vi "Periodic Tasks.vi"(8 "error in (no error)":errorcluster) -> ()   [LabVIEW 2016]
doc: "This VI runs in parallel to other tasks. It can contain as many user-defined periodic loops as you need. These can carry out PID or other sorts of timed response."
uses:
  Extra/Global_Var-RefNum/Global_Var_Other.vi
  Extra/General/ArbitorSpecializations/Arbitor_Int.vi
  Extra/General/ArbitorSpecializations/Arbitor_Float.vi
  Extra/General/ArbitorSpecializations/Arbitor_Bool.vi
  Extra/Sensors/ADI MXP IMU/ADIS16448_IMU.lvlib
  Extra/Sensors/PixyCam/PixyCam_LabVIEW.lvlib
panel:
  in  "Manual_Gate_Control":enum16{"Stop", "Catch", "Clamp", "Open"}(ring)
  in  "Gear_Beam_Break_Sensor_Triggered":bool
  in  "RailOffset":dbl=5.0 format="%#_13g"
  in  "UltrasonicPercent":dbl=0.2
  in  "MaxRange":dbl=27.0
  out "Distance":dbl=15.697590634880541
  in  "GearRailWantedPosition":dbl(slide)=5.0 scale=5.0..25.0
  in  "GearRailPID":T1={"proportional gain (Kc)"=0.2, "integral time (Ti, min)"=0.0, "derivative time (Td, min)"=0.0001} {"derivative time (Td, min)" format="%.3g"; "integral time (Ti, min)" format="%.3g"; "proportional gain (Kc)" format="%.3g"}
  in  "ResetGearCollect":bool
  in  "ResetGearPlacer":bool
  in  "StartGearPlace":bool
  in  "Place":bool
  in  "Collect":bool
  in  "Manual":bool=TRUE
  in  "StartGearCollect":bool
  out "GateReached":bool
  in  "Drive PID Gains":T1={"proportional gain (Kc)"=0.04, "integral time (Ti, min)"=0.025, "derivative time (Td, min)"=1e-05}
  out "IMU Angles Out":T2={"X Angle"=24.903333526419914, "Y Angle"=134.91891868799198, "Z Angle"=-74.78372775360221}
  # "1/24/17 (2014 Chassis)\nKc=0.015\nTi=5\nTd=0.0005\nTurns slowly, but well"
  # "2014 Chassis\nKc=0.09\nTi=0.9\nTd=0.001\nNot good for turning"
  # "2/12/17 (2017 Chassis)\nKc= 0.04\nTi=.025\nTd=1E-5\ndrives straight"
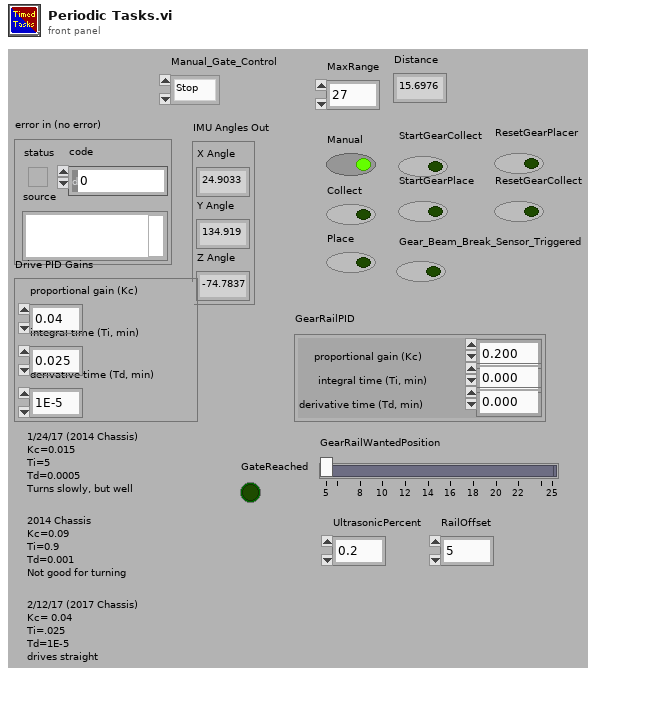
[diagram p1: front panel]
types:
  T1 = cluster{"proportional gain (Kc)":dbl, "integral time (Ti, min)":dbl, "derivative time (Td, min)":dbl}
  T2 = cluster{"X Angle":dbl, "Y Angle":dbl, "Z Angle":dbl}
  T3 = typedef "WPI_RobotDriveDevRef.ctl" = cluster{"DevStatus":errorcluster, "Motors[]":T4[], "Square Inputs":bool, "Max Output":dbl}
  T4 = typedef "WPI_MotorControlDeviceRef.ctl" = cluster{"DeviceStatus":errorcluster, "Type":T5, "PWM":cluster{"PWM Channel":T6, "DeadBand":T7}, "CAN":cluster{"Device Number":u8, "SetOutput VI Ref":variant, "GetOutput VI Ref":variant, "Enable VI Ref":variant, "Disable VI Ref":variant, "Data":variant}, "Invert":bool}
  T5 = typedef "WPI_MotorControlType.ctl" = enum16{"PWM", "CAN"}
  T6 = typedef "FPGA_DIOPWMChannel.ctl" = enum8{"PWM 0", "PWM 1", "PWM 2", "PWM 3", "PWM 4", "PWM 5", "PWM 6", "PWM 7", "PWM 8", "PWM 9", "PWM MXP 0", "PWM MXP 1", "PWM MXP 2", "PWM MXP 3", "PWM MXP 4", "PWM MXP 5", "PWM MXP 6", "PWM MXP 7", "PWM MXP 8", "PWM MXP 9", "Invalid"}
  T7 = typedef "WPI_PWMDeadband.ctl" = cluster{"Name":string, "maxPositivePwm":i32, "minPositivePwm":i32, "centerPwm":i32, "maxNegativePwm":i32, "minNegativePwm":i32, "angularRange":u16}
  T8 = typedef "PixyCam_LabVIEW.lvlib/PixyCam_DevRef.ctl" = cluster{"PixyCamDevRef_SPI":T9, "Communication Mode":T12, "Error":errorcluster}
  T9 = typedef "PixyCam_LabVIEW.lvlib/PixyCam_SPI_DevRef.ctl" = cluster{"SPIDevRef":T10, "Output Queue":refnum<queue>}
  T10 = typedef "WPI_SPIDevRef.ctl" = cluster{"DevStatus":errorcluster, "Handle":i32, "SPI Bus":T11}
  T11 = typedef "spi_bus.ctl" = enum16{"SPI On-Board, CS0", "SPI On-Board, CS1", "SPI On-Board, CS2", "SPI On-Board, CS3", "SPI MXP", "Invalid"}
  T12 = typedef "PixyCam_LabVIEW.lvlib/PixyCam_CommMode.ctl" = enum16{"SPI", "I2C", "UART", "Analog", "Digital"}
  T13 = typedef "ADIS16448_IMU.lvlib/ADI_IMU_ADIS16448_InterruptDevRef.ctl" = cluster{"ADI IMU DevRef":T14, "InterruptRef":T15}
  T14 = typedef "ADIS16448_IMU.lvlib/ADI_IMU_ADIS16448_IMUDevRef.ctl" = cluster{"DevStatus":errorcluster, "Handle":i32, "SPI Bus":T11, "Device Found":bool, "Device Ready":bool, "Yaw Axis":enum16{"X", "Y", "Z"}, "AHRS Algorithm":enum16{"Complementary", "Madgwick"}, "Serial":u16, "Lot ID 2":u16, "Lot ID 1":u16, "Product ID":u16}
  T15 = typedef "WPI_InterruptRef.ctl" = cluster{"DevStatus":errorcluster, "InterruptIndex":T16}
  T16 = typedef "FPGA_InterruptIndex.ctl" = enum8{"0", "1", "2", "3", "4", "5", "6", "7", "Invalid"}
  T17 = typedef "WPI_AnalogChannelDevRef.ctl" = cluster{"DevStatus":errorcluster, "Analog Channel":T18}
  T18 = typedef "FPGA_AIChannel.ctl" = enum8{"AI 0", "AI 1", "AI 2", "AI 3", "AI MXP 0", "AI MXP 1", "AI MXP 2", "AI MXP 3", "Invalid"}
  T19 = typedef "WPI_SonarMB1010DigitalDeviceRef.ctl" = cluster{"CounterDevRef":T20, "Scaling factor (s/in)":dbl}
  T20 = typedef "WPI_CounterDevRef.ctl" = cluster{"DevStatus":errorcluster, "CntIndex":T21}
  T21 = typedef "FPGA_CounterCtrSystemIndex.ctl" = enum8{"Ctr 0", "Ctr 1", "Ctr 2", "Ctr 3", "Ctr 4", "Ctr 5", "Ctr 6", "Ctr 7", "Invalid"}
  T22 = typedef "WPI_EncoderDevRef.ctl" = cluster{"DevStatus":errorcluster, "EncoderIndex":T23, "CounterIndex":T21, "DistancePerCount":dbl, "Decoding Type":T24}
  T23 = typedef "FPGA_EncoderIdx.ctl" = enum8{"Enc 0", "Enc 1", "Enc 2", "Enc 3", "Enc 4", "Enc 5", "Enc 6", "Enc 7", "Invalid"}
  T24 = typedef "WPI_EncoderType.ctl" = enum16{"1x", "2x", "4x"}
  T25 = typedef "WPI_DigitalInputDevRef.ctl" = cluster{"DevStatus":errorcluster, "DIO Channel":T26}
  T26 = typedef "FPGA_DIOChannel.ctl" = enum8{"DIO 0", "DIO 1", "DIO 2", "DIO 3", "DIO 4", "DIO 5", "DIO 6", "DIO 7", "DIO 8", "DIO 9", "DIO MXP 0", "DIO MXP 1", "DIO MXP 2", "DIO MXP 3", "DIO MXP 4", "DIO MXP 5", "DIO MXP 6", "DIO MXP 7", "DIO MXP 8", "DIO MXP 9", "DIO MXP 10", "DIO MXP 11", "DIO MXP 12", "DIO MXP 13", "DIO MXP 14", "DIO MXP 15", "SPI Port CS1", "SPI Port CS2", "SPI Port CS3", "SPI Port MISO", "SPI Port MOSI", "Invalid"}
  T27 = typedef "WPI_CompressorDevRef.ctl" = cluster{"DevStatus":errorcluster, "Pneumatics Control Module":u8}
  T28 = typedef "WPI_SolenoidDevRef.ctl" = cluster{"DevStatus":errorcluster, "Pneumatics Control Module":u8, "Forward Solenoid Channel":T29, "Reverse Solenoid Channel":T29}
  T29 = typedef "WPI_SolenoidChannel.ctl" = enum8{"Solenoid 0", "Solenoid 1", "Solenoid 2", "Solenoid 3", "Solenoid 4", "Solenoid 5", "Solenoid 6", "Solenoid 7", "Invalid"}
  T30 = cluster{"Motors":cluster{"Drive_Motor":cluster{"RobotDriveDevRef":T3, "error out":errorcluster}, "Shooter_Motor":cluster{"MotorControlDevRef":T4, "error out":errorcluster}, "Shooter_Feeder_Motor":cluster{"MotorControlDevRef":T4, "error out":errorcluster}, "Intake_Motor_1":cluster{"MotorControlDevRef":T4, "error out":errorcluster}, "Gear_Gate_Motor":cluster{"MotorControlDevRef":T4, "error out":errorcluster}, "Climber_Motor":cluster{"MotorControlDevRef":T4, "error out":errorcluster}, "Shooter_Turret_Motor":cluster{"MotorControlDevRef":T4, "error out":errorcluster}, "Top_Shooter_Feeder_Motor":cluster{"MotorControlDevRef":T4, "error out":errorcluster}, "Gear_Rail_Motor":cluster{"MotorControlDevRef":T4, "error out":errorcluster}}, "Sensors":cluster{"PixyCam":cluster{"PixyCamDevRef Out":T8, "error out":errorcluster}, "IMU":cluster{"ADI IMU Interrupt DevRef":T13, "error out":errorcluster}, "Pots":cluster{"Gear_Gate_Pot":cluster{"AIDeviceRef":T17, "error out":errorcluster}, "Gear_Rail_Pot":cluster{"AIDeviceRef":T17, "error out":errorcluster}, "Turret_Pot":cluster{"AIDeviceRef":T17, "error out":errorcluster}}, "Ultrasonics":cluster{"Gear_Peg_Ultrasonic":cluster{"SonarMB1010DigitalDevRef":T19, "error out":errorcluster}}, "Encoders":cluster{"Drive_Encoder":cluster{"EncoderDevRef":T22, "error out":errorcluster}, "Shooter_Encoder":cluster{"EncoderDevRef":T22, "error out":errorcluster}}, "DIOs":cluster{"Gear_Beambreak":cluster{"DigitalInputDevRef":T25, "error out":errorcluster}, "Ball_Beambreak":cluster{"DigitalInputDevRef":T25, "error out":errorcluster}}}, "Pneumatics":cluster{"Compressor":cluster{"CompressorDevRef":T27, "error out":errorcluster}, "Gear_Pusher":cluster{"SolenoidDevRef":T28, "error out":errorcluster}, "Shifters":cluster{"SolenoidDevRef":T28, "error out":errorcluster}, "Gear_Chute":cluster{"SolenoidDevRef":T28, "error out":errorcluster}}}
  T31 = cluster{"Joystick_1":cluster{"Joystick_Unassigned":dbl, "Joystick_F/B":dbl, "Joystick_L/R_Turn":dbl, "Joysick_Unassigned":dbl, "Joystick_Unassigned":dbl, "Joystick_Gearpusher":bool, "Joystick_Climb":bool, "Joystick_Intake":bool, "Joystick_Place_Gear":bool, "Joystick_DriveStraight":bool, "Joysick_Shoot":bool, "Joystick_Shift":bool, "Joystick_Aim":bool, "Joysick_Lightshow":bool}, "Joystick_2":cluster{"Joystick_GearRail_R/L":dbl, "Joystick_Climb_UpDown":dbl, "Joystick_Turret_L/R":dbl, "Joystick_Unassigned":dbl, "Joystick_BotFeed_F":bool, "Joystick_BotFeed_B":bool, "Joystick_GateOpen":bool, "Joystick_GateClose":bool, "Joystick_GateClamp":bool, "Joystick_Intake_B":bool, "Joystick_Feed_F":bool, "Joysitick_Feed_B":bool, "Joystick_GearChute":bool, "Joystick_Unassigned":dbl}}
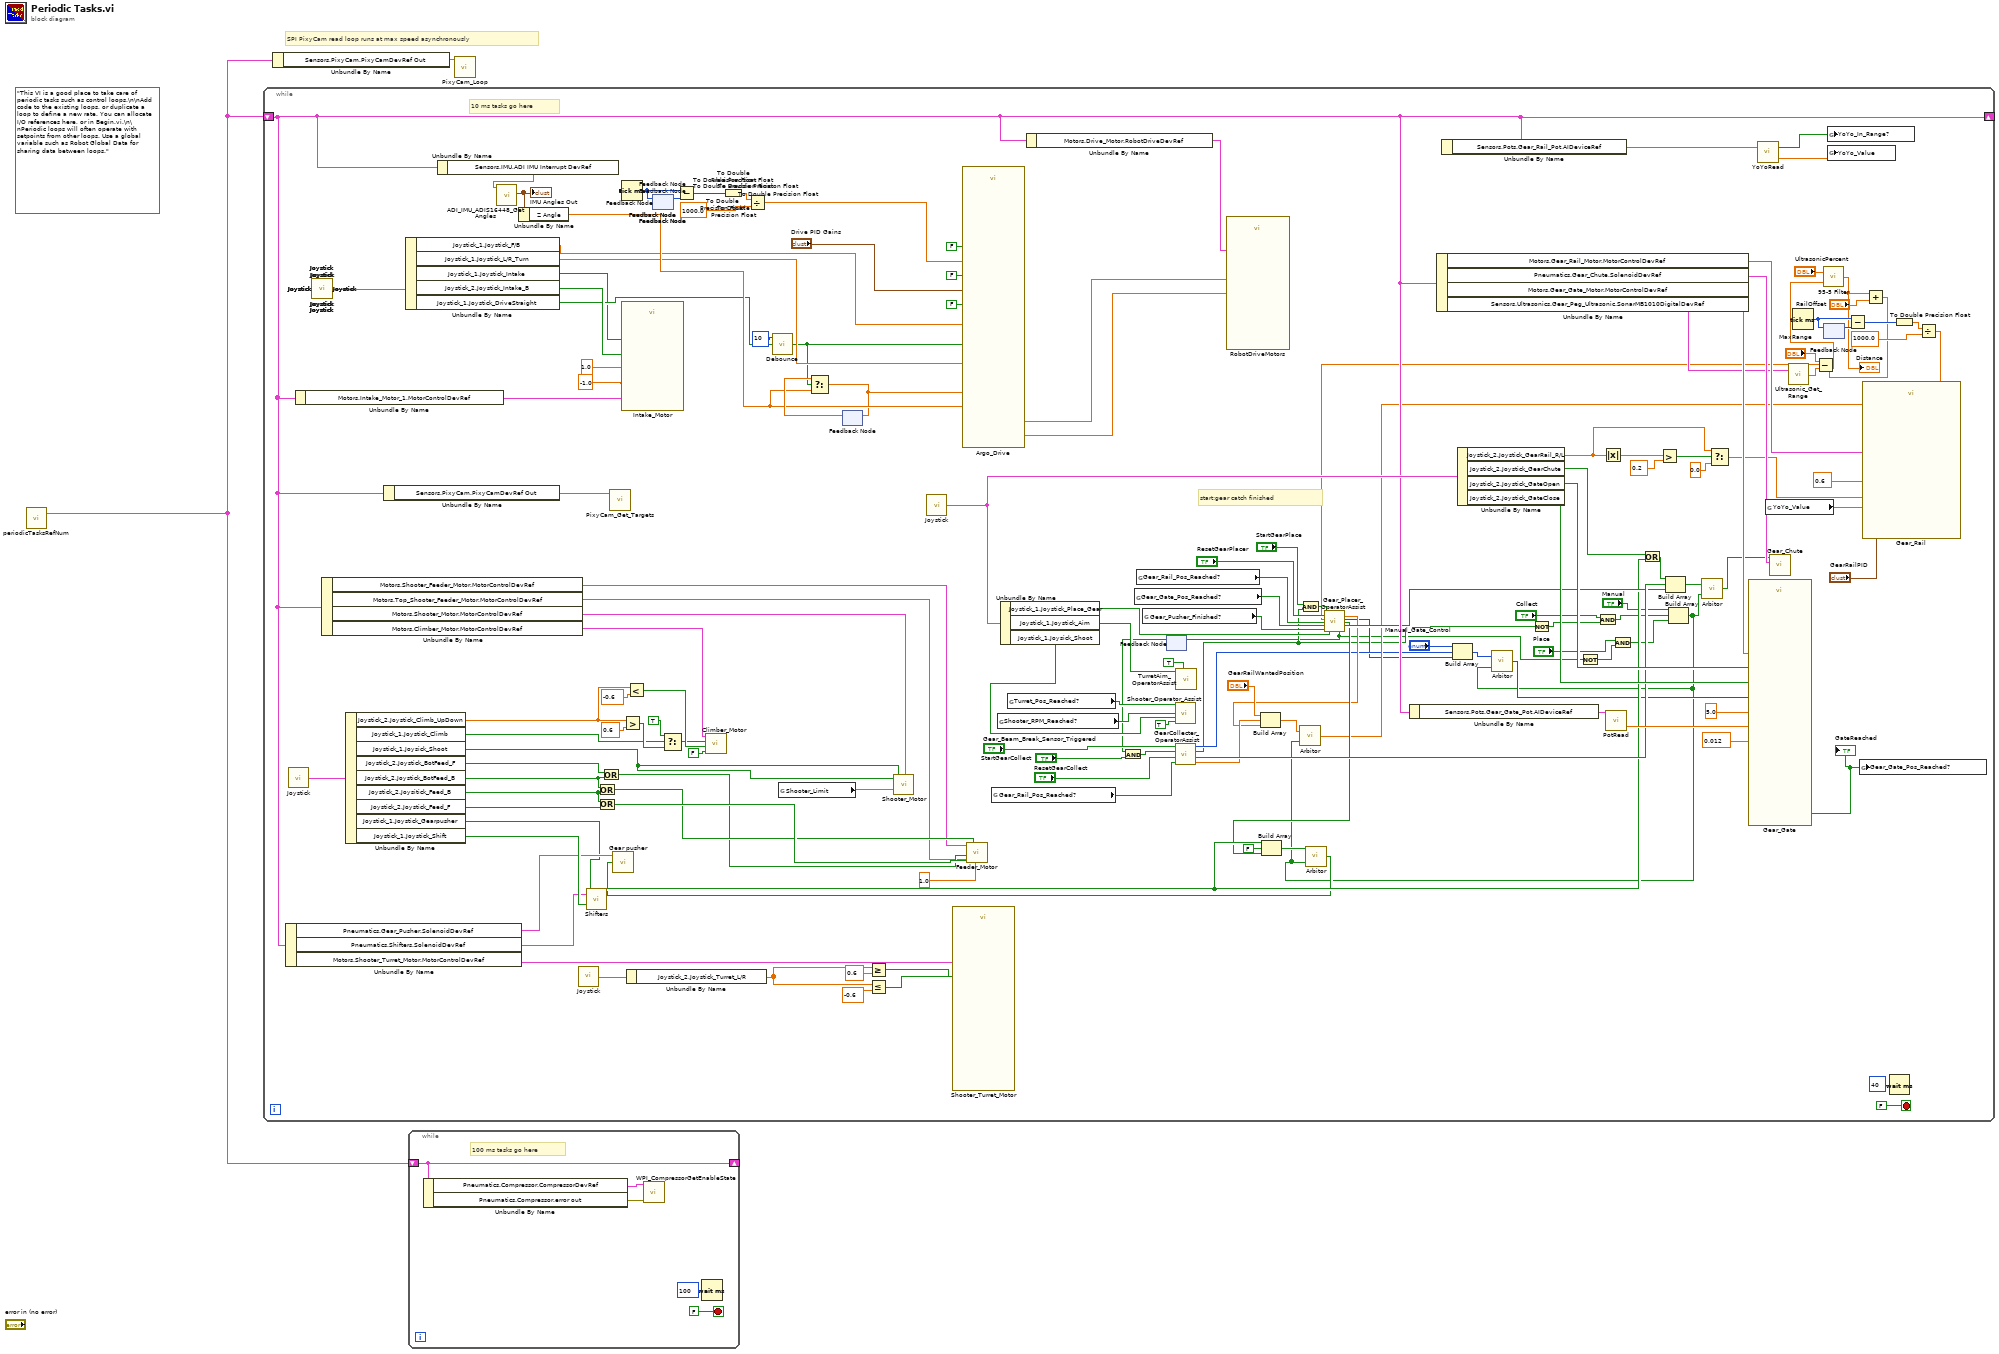
[diagram p0: block diagram]
diagram:
  (unwired) "This VI is a good place to take care of periodic tasks such as control loops.\n\nAdd code to the existing loops, or duplicate a loop to define a new rate. You can allocate I/O references here, or in Begin.vi.\n\nPeriodic loops will often operate with setpoints from other loops. Use a global variable such as Robot Global Data for sharing data between loops."
  # "SPI PixyCam read loop runs at max speed asynchronously"
  n1 = call "periodicTasksRefNum.vi"() -> ("RefNums"=w2:T30)  [unwired: 3 in]
  n2 = while {
    shift-right: [w90] -> _
    shift-left: w2 -> [w90]
    stop <- FALSE stop-if-true
    # "start:gear catch finished"
    # "10 ms tasks go here"
    n3 = Unbundle By Name(w90) -> ("Pneumatics.Gear_Pusher.SolenoidDevRef"=w115:T28, "Pneumatics.Shifters.SolenoidDevRef"=w114:T28, "Motors.Shooter_Turret_Motor.MotorControlDevRef"=w113:T4)
    n4 = call "Joystick.vi"() -> ("Joystick"=w121:T31)  [unwired: 1 in]
    n5 = Unbundle By Name(w90) -> ("Motors.Intake_Motor_1.MotorControlDevRef"=w125:T4)
    n6 = call "Joystick.vi"() -> ()  [unwired: 1 in, 1 out]
    n7 = call "Joystick.vi"() -> ()  [unwired: 1 in, 1 out]
    n8 = call "Joystick.vi"() -> ()  [unwired: 1 in, 1 out]
    n9 = call "Joystick.vi"() -> ()  [unwired: 1 in, 1 out]
    n10 = call "Joystick.vi"() -> ()  [unwired: 1 in, 1 out]
    n11 = call "Joystick.vi"() -> ()  [unwired: 1 in, 1 out]
    n12 = call "Joystick.vi"() -> ()  [unwired: 1 in, 1 out]
    n13 = call "Joystick.vi"() -> ()  [unwired: 1 in, 1 out]
    n14 = call "Joystick.vi"() -> ()  [unwired: 1 in, 1 out]
    n15 = call "Joystick.vi"() -> ()  [unwired: 1 in, 1 out]
    n16 = call "Joystick.vi"() -> ()  [unwired: 1 in, 1 out]
    n17 = call "Joystick.vi"() -> ()  [unwired: 1 in, 1 out]
    n18 = call "Joystick.vi"() -> ()  [unwired: 1 in, 1 out]
    n19 = call "Joystick.vi"() -> ()  [unwired: 1 in, 1 out]
    n20 = call "Joystick.vi"() -> ()  [unwired: 1 in, 1 out]
    n21 = call "Joystick.vi"() -> ()  [unwired: 1 in, 1 out]
    n22 = call "Joystick.vi"() -> ()  [unwired: 1 in, 1 out]
    n23 = call "Joystick.vi"() -> ()  [unwired: 1 in, 1 out]
    n24 = call "Joystick.vi"() -> ()  [unwired: 1 in, 1 out]
    n25 = call "Joystick.vi"() -> ()  [unwired: 1 in, 1 out]
    n26 = call "Joystick.vi"() -> ()  [unwired: 1 in, 1 out]
    n27 = call "Joystick.vi"() -> ("Joystick"=w136:T31)  [unwired: 1 in]
    n28 = Unbundle By Name(w90) -> ("Motors.Shooter_Feeder_Motor.MotorControlDevRef"=w116:T4, "Motors.Top_Shooter_Feeder_Motor.MotorControlDevRef"=w117:T4, "Motors.Shooter_Motor.MotorControlDevRef"=w118:T4, "Motors.Climber_Motor.MotorControlDevRef"=w119:T4)
    n29 = Unbundle By Name(w121) -> ("Joystick_2.Joystick_Climb_UpDown"=w144:dbl, "Joystick_1.Joystick_Climb"=w143:bool, "Joystick_1.Joysick_Shoot"=w142:bool, "Joystick_2.Joystick_BotFeed_F"=w111:bool, "Joystick_2.Joystick_BotFeed_B"=w112:bool, "Joystick_2.Joysitick_Feed_B"=w137:bool, "Joystick_2.Joystick_Feed_F"=w141:bool, "Joystick_1.Joystick_Gearpusher"=w34:bool, "Joystick_1.Joystick_Shift"=w145:bool)
    n30 = Unbundle By Name(w90) -> ("Sensors.PixyCam.PixyCamDevRef Out"=w108:T8)
    n31 = Unbundle By Name(w136) -> ("Joystick_1.Joystick_F/B"=w160:dbl, "Joystick_1.Joystick_L/R_Turn"=w159:dbl, "Joystick_1.Joystick_Intake"=w152:bool, "Joystick_2.Joystick_Intake_B"=w158:bool, "Joystick_1.Joystick_DriveStraight"=w157:bool)
    n32 = Unbundle By Name(w90) -> ("Sensors.IMU.ADI IMU Interrupt DevRef"=w174:T13)
    n33 = call "ADI_IMU_ADIS16448_Get Angles.vi"("ADI IMU Interrupt DevRef"=w174) -> ("IMU Angles Out"=w167:T2)  [unwired: 7 in, 3 out]
    "IMU Angles Out" <- w167
    n34 = Unbundle By Name(w167) -> ("Z Angle"=w163:dbl)
    n35 = call "Joystick.vi"() -> ("Joystick"=w110:T31)  [unwired: 1 in]
    n36 = call "Shifters.vi"("High Gear"=w145, "ShifterDevRef"=w114) -> ()  [unwired: 1 in]
    n37 = Or(x=w112, y=w137) -> (x .or. y?=w139:bool)
    n38 = Or(x=w137, y=w141) -> (x .or. y?=w140:bool)
    n39 = Or(x=w111, y=w112) -> (x .or. y?=w138:bool)
    n40 = call "PixyCam_Get_Targets.vi"("PixyCamDevRef"=w108) -> ()  [unwired: 4 in, 3 out]
    n41 = call "Intake_Motor.vi"("Forward_Button_Pushed?"=w152, "Reverse_Button_Pushed?"=w158, "MotorControlDevRef"=w125, "Intake_Motor_Limit_Forward"=1.0, "Intake_Motor_Limit_Backward"=-1.0) -> ()  [unwired: 1 in]
    n42 = Tick Count (ms)() -> (millisecond timer value=w53:u32)
    n43 = Tick Count (ms)() -> (millisecond timer value=w56:u32)
    n44 = Tick Count (ms)() -> (millisecond timer value=w63:u32)
    n45 = Tick Count (ms)() -> (millisecond timer value=w66:u32)
    n46 = Tick Count (ms)() -> (millisecond timer value=w71:u32)
    n47 = Tick Count (ms)() -> (millisecond timer value=w76:u32)
    n48 = Tick Count (ms)() -> (millisecond timer value=w172:u32)
    n49 = Greater?(x=w144, y=0.6) -> (0:w147:bool)
    n50 = Less?(x=w144, y=-0.6) -> (x < y?=w149:bool)
    n51 = Unbundle By Name(w110) -> ("Joystick_2.Joystick_Turret_L/R"=w109:dbl)
    n52 = feedback #1() -> (w54:u32)  [unwired: 1 in]
    n53 = feedback-in #1(w53) -> ()
    n54 = feedback #2() -> (w55:u32)  [unwired: 1 in]
    n55 = feedback-in #2(w56) -> ()
    n56 = feedback #3() -> (w64:u32)  [unwired: 1 in]
    n57 = feedback-in #3(w63) -> ()
    n58 = feedback #4() -> (w65:u32)  [unwired: 1 in]
    n59 = feedback-in #4(w66) -> ()
    n60 = feedback #5() -> (w70:u32)  [unwired: 1 in]
    n61 = feedback-in #5(w71) -> ()
    n62 = feedback #6() -> (w75:u32)  [unwired: 1 in]
    n63 = feedback-in #6(w76) -> ()
    n64 = feedback-in #7(w172) -> ()
    n65 = feedback #7() -> (w173:u32)  [unwired: 1 in]
    n66 = Select(t=TRUE, s=w143, f=w147) -> (s? t:f=w146:bool)
    n67 = Subtract(x=w53, y=w54) -> (x-y=w51:u32)
    n68 = Subtract(x=w56, y=w55) -> (x-y=w58:u32)
    n69 = Subtract(x=w63, y=w64) -> (x-y=w61:u32)
    n70 = Subtract(x=w66, y=w65) -> (x-y=w68:u32)
    n71 = Subtract(x=w71, y=w70) -> (x-y=w73:u32)
    n72 = Subtract(x=w76, y=w75) -> (x-y=w78:u32)
    n73 = Subtract(x=w172, y=w173) -> (x-y=w170:u32)
    n74 = call "Climber_Motor.vi"("Invert?"=FALSE, "Climb_Down?"=w149, "Climb_Up?"=w146, "MotorControlDevRef"=w119) -> ()  [unwired: 8 in]
    n75 = To Double Precision Float(number=w51) -> (double precision float=w50:dbl)
    n76 = To Double Precision Float(number=w58) -> (double precision float=w59:dbl)
    n77 = To Double Precision Float(number=w61) -> (double precision float=w60:dbl)
    n78 = To Double Precision Float(number=w68) -> (double precision float=w69:dbl)
    n79 = To Double Precision Float(number=w73) -> (double precision float=w74:dbl)
    n80 = To Double Precision Float(number=w78) -> (double precision float=w79:dbl)
    n81 = To Double Precision Float(number=w170) -> (double precision float=w169:dbl)
    n82 = Divide(x=w50, y=1000.0) -> ()  [unwired: 1 out]
    n83 = Divide(x=w59, y=1000.0) -> ()  [unwired: 1 out]
    n84 = Divide(x=w60, y=1000.0) -> ()  [unwired: 1 out]
    n85 = Divide(x=w69, y=1000.0) -> ()  [unwired: 1 out]
    n86 = Divide(x=w74, y=1000.0) -> ()  [unwired: 1 out]
    n87 = Divide(x=w79, y=1000.0) -> ()  [unwired: 1 out]
    n88 = Divide(x=w169, y=1000.0) -> (x/y=w168:dbl)
    n89 = call "Debounce.vi"("Input"=w157, "Num samples"=10) -> ("Output"=w96:bool)  [unwired: 1 in]
    n90 = global read "Global_Var_Other.vi" "Shooter_Limit"() -> (w177:dbl)
    n91 = feedback #8() -> (w164:dbl)  [unwired: 1 in]
    n92 = Select(t=w164, s=w96, f=w163) -> (s? t:f=w95:dbl)
    n93 = feedback-in #8(w95) -> ()
    n94 = Greater Or Equal?(x=w109, y=0.6) -> (x >= y?=w156:bool)
    n95 = Less Or Equal?(x=w109, y=-0.6) -> (x <= y?=w155:bool)
    n96 = call "Shooter_Motor.vi"("MotorControlDevRef"=w118, "Shooter_Auto?"=w142, "dt_In_PID"=w177, "Shooter_Forward?"=w142) -> ()  [unwired: 14 in, 2 out]
    n97 = call "Joystick.vi"() -> ("Joystick"=w120:T31)  [unwired: 1 in]
    n98 = call "Shooter_Turret_Motor.vi"("MotorControlDevRef"=w113, "Turret_Clockwise?"=w156, "Turret_Counterclockwise?"=w155) -> ()  [unwired: 24 in, 1 out]
    n99 = call "Argo_Drive.vi"("Speed_Main"=w160, "Turning_PID_Enable"=w96, "PID Gains"="Drive PID Gains", "Turning_Main"=w159, "Auto_Enable"=FALSE, "High_Gear"=FALSE, "Quick_Turn"=FALSE, "Turning_Setpoint"=w95, "dt (s)"=w168, "Yaw"=w163) -> ("Left_Motor"=w183:dbl, "Right_Motor"=w182:dbl)  [unwired: 8 in]
    n100 = call "Feeder_Motor.vi"("Shooter_Feeder_Motor_Limit"=1.0, "Invert?"=w139, "RunTopRoller"=w140, "Feeder_Button_Pressed?"=w138, "TopMotorDevRef"=w117, "BottomMotorDevRef"=w116) -> ()  [unwired: 1 out]
    n101 = global read "Global_Var_Other.vi" "Gear_Rail_Pos_Reached?"() -> (w28:bool)
    n102 = global read "Global_Var_Other.vi" "Shooter_RPM_Reached?"() -> (w129:bool)
    n103 = Unbundle By Name(w120) -> ("Joystick_1.Joystick_Place_Gear"=w132:bool, "Joystick_1.Joystick_Aim"=w131:bool, "Joystick_1.Joysick_Shoot"=w128:bool)
    n104 = global read "Global_Var_Other.vi" "Turret_Pos_Reached?"() -> (w130:bool)
    n105 = Unbundle By Name(w90) -> ("Motors.Drive_Motor.RobotDriveDevRef"=w184:T3)
    n106 = global read "Global_Var_Other.vi" "Gear_Gate_Pos_Reached?"() -> (w134:bool)
    n107 = global read "Global_Var_Other.vi" "Gear_Rail_Pos_Reached?"() -> (w135:bool)
    n108 = global read "Global_Var_Other.vi" "Gear_Pusher_Finished?"() -> (w133:bool)
    n109 = feedback #9() -> (w11:bool)  [unwired: 1 in]
    n110 = And(x=w11, y="StartGearCollect") -> (x .and. y?=w13:bool)
    n111 = call "Shooter_Operator_Assist.vi"("Turret Aimed"=w130, "Shooter Motor Speed Good"=w129, "Shoot Command"=w128, "Start"=TRUE) -> ()  [unwired: 8 in, 4 out]
    n112 = call "GearCollecter_OperatorAssist.vi"("CarriageReturned"=w28, "Manual_Overide"="ResetGearCollect", "Start"=w13, "Gear_Beam_Break_Sensor_Triggered"="Gear_Beam_Break_Sensor_Triggered") -> ("Gear_Rail_Position"=w25:dbl, "GearChuteExtend"=w85:bool, "Catch_Complete?"=w7:bool, "Gate_Pos"=w21:enum16{"Stop", "Catch", "Clamp", "Open"})
    n113 = call "TurretAim_OperatorAssist.vi"("Start"=TRUE, "Reacquire"=w131) -> ()  [unwired: 5 in, 1 out]
    n114 = call "RobotDriveMotors.vi"("RightSpeed"=w182, "LeftSpeed"=w183, "RobotDriveDevRef"=w184) -> ()  [unwired: 6 in, 3 out]
    n115 = And(x="StartGearPlace", y=w7) -> (x .and. y?=w15:bool)
    n116 = Unbundle By Name(w90) -> ("Sensors.Pots.Gear_Gate_Pot.AIDeviceRef"=w89:T17)
    n117 = Unbundle By Name(w90) -> ("Motors.Gear_Rail_Motor.MotorControlDevRef"=w124:T4, "Pneumatics.Gear_Chute.SolenoidDevRef"=w123:T28, "Motors.Gear_Gate_Motor.MotorControlDevRef"=w122:T4, "Sensors.Ultrasonics.Gear_Peg_Ultrasonic.SonarMB1010DigitalDevRef"=w43:T19)
    n118 = Unbundle By Name(w90) -> ("Sensors.Pots.Gear_Rail_Pot.AIDeviceRef"=w161:T17)
    n119 = Unbundle By Name(w120) -> ("Joystick_2.Joystick_GearRail_R/L"=w100:dbl, "Joystick_2.Joystick_GearChute"=w104:bool, "Joystick_2.Joystick_GateOpen"=w94:bool, "Joystick_2.Joystick_GateClose"=w93:bool)
    n120 = Not(x=w7) -> (.not. x?=w8:bool)
    n121 = And(x="Collect", y=w8) -> (x .and. y?=w9:bool)
    n122 = Absolute Value(x=w100) -> (abs(x)=w103:dbl)
    n123 = call "PotRead.vi"("PotDevRef"=w89) -> ("Pot"=w88:dbl)  [unwired: 4 in, 1 out]
    n124 = Or(x=w104, y=w34) -> (x .or. y?=w86:bool)
    n125 = Greater?(x=w103, y=0.2) -> (0:w101:bool)
    n126 = Select(t=w100, s=w101, f=0.0) -> (s? t:f=w98:dbl)
    n127 = call "YoYoRead.vi"("YoYoDevRef"=w161) -> ("YoYo"=w107:dbl, "In_Range?"=w106:bool)  [unwired: 1 in]
    n128 = global read "Global_Var_Other.vi" "YoYo_Value"() -> (w105:dbl)
    n129 = call "Ultrasonic_Get_Range.vi"("SonarMB1010DigitalDevRef"=w43) -> ("Range"=w42:dbl)  [unwired: 2 in, 2 out]
    n130 = Tick Count (ms)() -> (millisecond timer value=w46:u32)
    n131 = Subtract(x="MaxRange", y=w42) -> (x-y=w40:dbl)
    n132 = call "95-5 Filter.vi"("In"=w40, "Percent"="UltrasonicPercent") -> ("Out"=w38:dbl)
    "Distance" <- w38
    n133 = feedback #10() -> (w45:u32)  [unwired: 1 in]
    n134 = feedback-in #10(w46) -> ()
    n135 = global write "Global_Var_Other.vi" "YoYo_In_Range?"(w106) -> ()
    n136 = global write "Global_Var_Other.vi" "YoYo_Value"(w107) -> ()
    n137 = Subtract(x=w46, y=w45) -> (x-y=w48:u32)
    n138 = Add(x=w38, y="RailOffset") -> (x+y=w36:dbl)
    n139 = call "Gear_Placer_OperatorAssist.vi"("Start?"=w15, "Reset?"="ResetGearPlacer", "Ultrasonic"=w36, "Rail_Finished?"=w135, "Gate_Finished?"=w134, "Gear_Pusher_Finished?"=w133, "Place_Gear?"=w132) -> ("Place_Complete?"=w3:bool, "Rail_Target_Position"=w23:dbl, "Gate_Pos"=w18:enum16{"Stop", "Catch", "Clamp", "Open"}, "Gear_Pusher_Extend?"=w31:bool, "Gear_Chute_Extend?"=w35:bool)  [unwired: 6 in, 2 out]
    n140 = feedback-in #9(w3) -> ()
    n141 = Build Array("GearRailWantedPosition", w25, w23) -> (w26:dbl[])
    n142 = Build Array(w34, FALSE, w31) -> (w33:bool[])
    n143 = Build Array("Manual_Gate_Control", w21, w18) -> (w20:enum16{"Stop", "Catch", "Clamp", "Open"}[])
    n144 = Not(x=w3) -> (.not. x?=w4:bool)
    n145 = And(x="Place", y=w4) -> (x .and. y?=w5:bool)
    n146 = Build Array(w86, w85, w35) -> (w84:bool[])
    n147 = Build Array("Manual", w9, w5) -> (w16:bool[])
    n148 = call-poly "Arbitor.vi"("Selector Array"=w16, "Input Array"=w26) -> ("Arbitrated Output"=w22:dbl)
    n149 = call-poly "Arbitor.vi"("Selector Array"=w16, "Input Array"=w33) -> ("Arbitrated Output"=w29:bool)
    n150 = call "Gear pusher.vi"("Extend"=w29, "Cylinder_Devref"=w115) -> ()  [unwired: 3 in]
    n151 = call-poly "Arbitor.vi"("Selector Array"=w16, "Input Array"=w20) -> ("Arbitrated Output"=w19:i32)
    n152 = call-poly "Arbitor.vi"("Selector Array"=w16, "Input Array"=w84) -> ("Arbitrated Output"=w83:bool)
    n153 = call "Gear_Gate.vi"("MotorControlDevRef"=w122, "Open_Button_Pressed?"=w94, "Close_Button_Pressed?"=w93, "Potentiometer_Input"=w88, "Gate_Pos"=w19, "Acceptable_Range"=5.0, "Scale_Factor"=0.012) -> ("Reached"=w92:bool)  [unwired: 12 in]
    "GateReached" <- w92
    n154 = call "Gear_Chute.vi"("SolenoidDevRef"=w123, "Extend?"=w83) -> ()  [unwired: 10 in]
    n155 = global write "Global_Var_Other.vi" "Gear_Gate_Pos_Reached?"(w92) -> ()
    n156 = Wait (ms)(milliseconds to wait=u32 40) -> ()  [unwired: 1 out]
    n157 = To Double Precision Float(number=w48) -> (double precision float=w49:dbl)
    n158 = Divide(x=w49, y=1000.0) -> (x/y=w44:dbl)
    n159 = call "Gear_Rail.vi"("MotorControlDevRef"=w124, "dt_In_PID"=w44, "Potentiometer_Input"=w105, "Potentiometer_WantedPos"=w22, "Motor_Input"=w98, "Motor_Limit"=0.6, "PID gains"="GearRailPID") -> ()  [unwired: 20 in, 1 out]
  }
  n160 = Unbundle By Name(w2) -> ("Sensors.PixyCam.PixyCamDevRef Out"=w1:T8)
  n161 = while {
    shift-right: [w189] -> _
    shift-left: w2 -> [w189]
    stop <- FALSE stop-if-true
    # "100 ms tasks go here"
    n162 = Unbundle By Name(w189) -> ("Pneumatics.Compressor.CompressorDevRef"=w188:T27, "Pneumatics.Compressor.error out"=w187:errorcluster)
    n163 = call <vilib>:"WPI_CompressorGetEnableState.vi"("error in (no error)"=w187, "CompressorDevRef"=w188) -> ()  [unwired: 6 in, 4 out]
    n164 = Wait (ms)(milliseconds to wait=u32 100) -> ()  [unwired: 1 out]
  }
  n165 = call "PixyCam_Loop.vi"("PixyCamDevRef"=w1) -> ()  [unwired: 5 in, 2 out]
